vi "PH_ImageOperator.FF ThresholdImage.vi"(0 "Image":T1, 2 "threshold":dbl=0.12999999523162842 min=0.0 max=1.0, 5 "error in (no error)":errorcluster) -> (14 "Image Dst Out":T1, 19 "error out":errorcluster)   [LabVIEW 2014, in "PH_ImageOperator.lvlib"]
doc: "This VI generates a \"binary\" image with pixels values of either 1 or 0 based on a given relative threshold value (0.0-1.0). NOTE: This VI assumes an 8bit picture type (max. pixel value is hard-coded as 255)."
uses:
  PH_ImageOperator.lvlib
  <vilib>/vision/Image Controls.llb/IMAQ Image.ctl
  <vilib>/vision/NI_Vision_Development_Module.lvlib
panel:
  in  "Range":cluster{"Lower value":sgl, "Upper value":sgl}={"Lower value"=128.0, "Upper value"=255.0} {"Upper value" format="%.2f"; "Lower value" format="%.2f"}
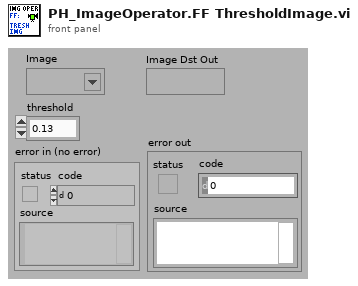
[diagram p1: front panel]
types:
  T1 = typedef "IMAQ Image.ctl" = refnum<image>
  T2 = cluster{"histogram":u32[], "Minimal Value":sgl, "Maximal Value":sgl, "Starting Value":sgl, "Interval Width":sgl, "Mean Value":sgl, "Standard  Variation":sgl, "Area (pixels)":i32}
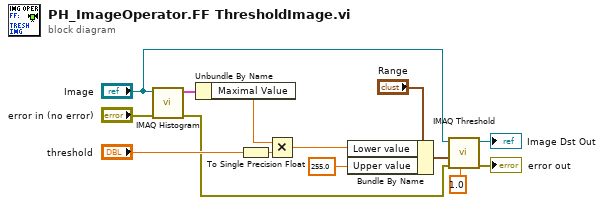
[diagram p0: block diagram]
diagram:
  n1 = call "IMAQ Histogram"("error in (no error)"="error in (no error)", "Image"="Image") -> ("error out"=w1:errorcluster, "Histogram Report"=w10:T2)  [unwired: 8 in]
  n2 = Unbundle By Name(w10) -> ("Maximal Value"=w12:sgl)
  n3 = To Single Precision Float(number="threshold") -> (single precision float=w2:sgl)
  n4 = Multiply(x=w12, y=w2) -> (x*y=w11:sgl)
  n5 = Bundle By Name(cluster="Range", "Lower value"=w11, "Upper value"=sgl 255.0) -> (w5:cluster{"Lower value":sgl, "Upper value":sgl})
  n6 = call "IMAQ Threshold"("Replace Value"=sgl 1.0, "error in (no error)"=w1, "Range"=w5, "Image Src"="Image") -> ("error out"=→"error out":errorcluster, "Image Dst Out"=→"Image Dst Out":T1)  [unwired: 6 in]
